vi "get tag counts.vi"(11 "data dictionary in":refnum<class "data dictionary.lvclass">) -> (2 "counts":T1[](array[typedef]), 3 "data dictionary out":refnum<class "data dictionary.lvclass">)   [LabVIEW 2013, in "tag bus.lvlib" / "data dictionary.lvclass"]
doc: "Gets the constitution of the data table, returning an array of types and the associated tag count of each type. If the dictionary is empty, this returns an empty array."
uses:
  data dictionary.lvclass
  table/allocation specification.ctl
  tag/Data Type.ctl
  data dictionary.lvclass/data dictionary.ctl
  tag/count types.vi
  tag/index to type.vi
  tag/tag descriptor.lvclass
  table/data table.lvlib
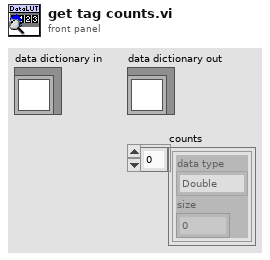
[diagram p1: front panel]
types:
  T1 = typedef "tag bus.lvlib/data table.lvlib/allocation specification.ctl" = cluster{"data type":T2, "size":i32}
  T2 = typedef "tag bus.lvlib/tag descriptor.lvclass/Data Type.ctl" = enum16{"Double", "Single", "I64", "I32", "I16", "I8", "U64", "U32", "U16", "U8", "Boolean", "String", "Array of Double", "Array of Single", "Array of I64", "Array of I32", "Array of I16", "Array of I8", "Array of U64", "Array of U32", "Array of U16", "Array of U8", "Array of Boolean", "Array of String"}
  T3 = typedef "tag bus.lvlib/binary search.lvlib/sorted list.ctl" = cluster{"sorted strings":string[], "sorted indices":i32[]}
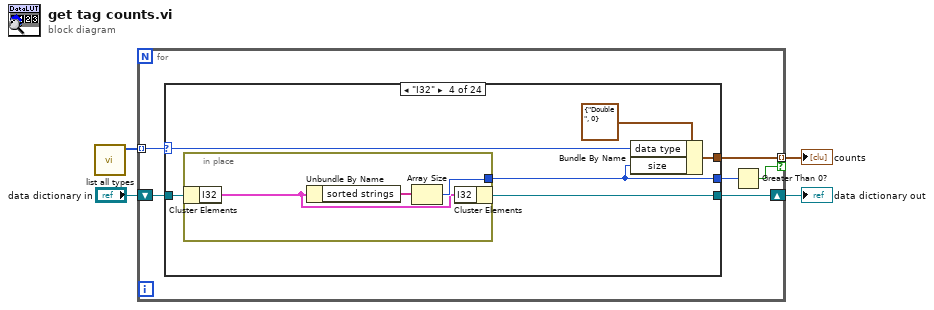
[diagram p0: block diagram]
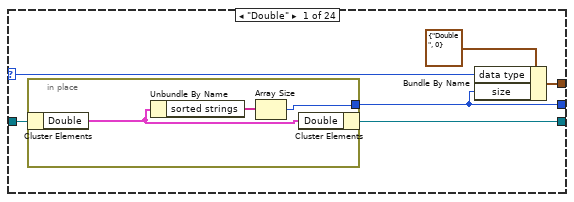
[diagram p2: hidden frame]
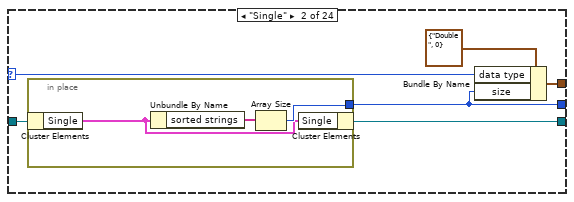
[diagram p3: hidden frame]
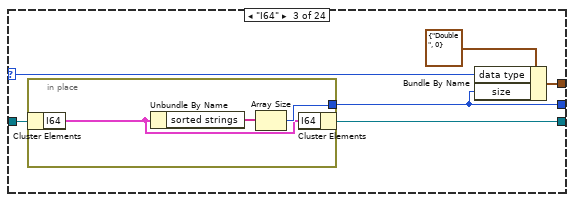
[diagram p4: hidden frame]
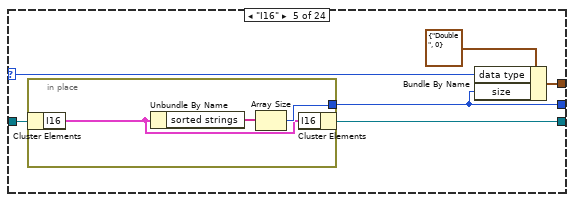
[diagram p5: hidden frame]
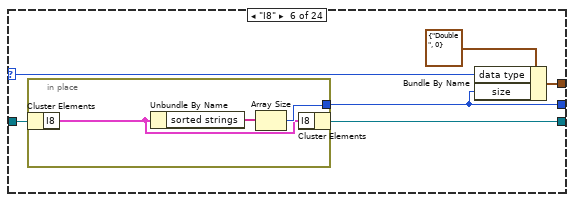
[diagram p6: hidden frame]
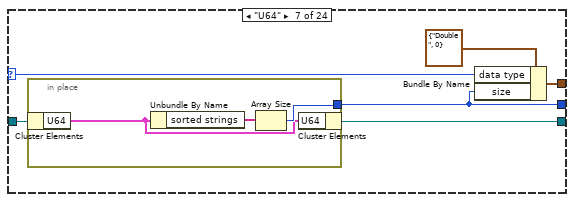
[diagram p7: hidden frame]
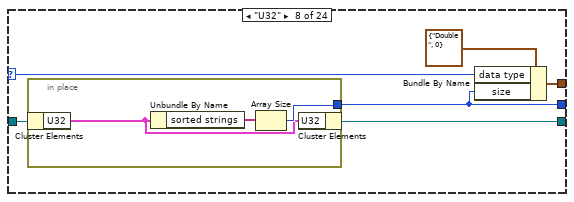
[diagram p8: hidden frame]
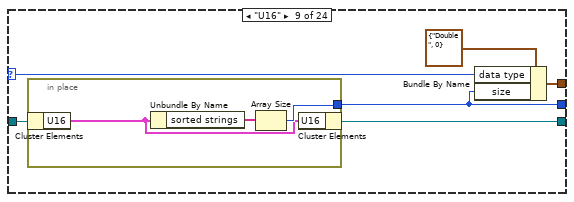
[diagram p9: hidden frame]
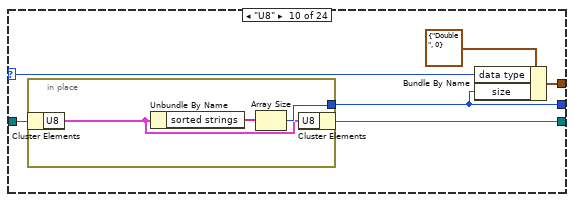
[diagram p10: hidden frame]
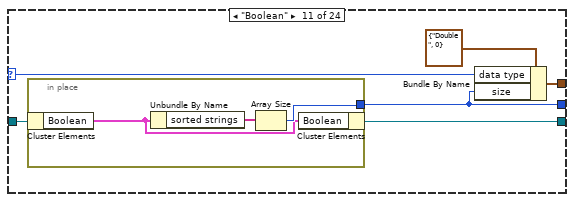
[diagram p11: hidden frame]
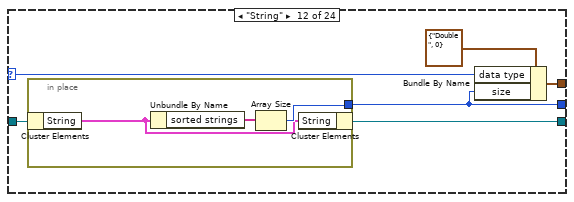
[diagram p12: hidden frame]
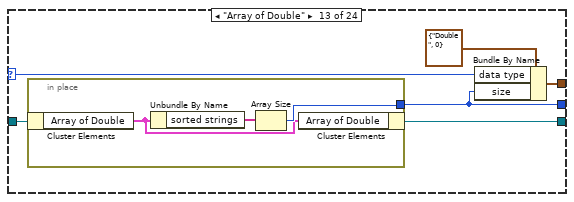
[diagram p13: hidden frame]
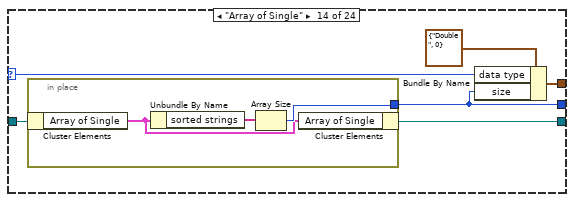
[diagram p14: hidden frame]
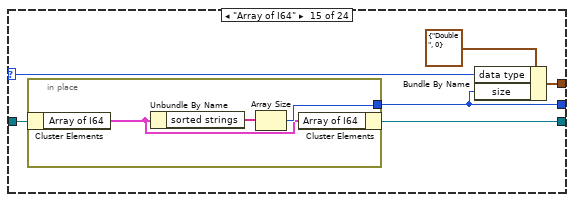
[diagram p15: hidden frame]
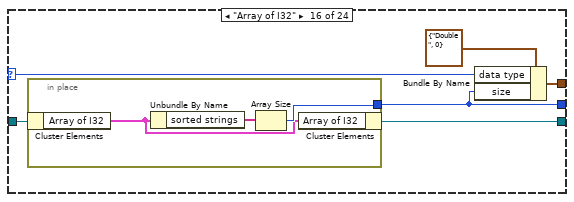
[diagram p16: hidden frame]
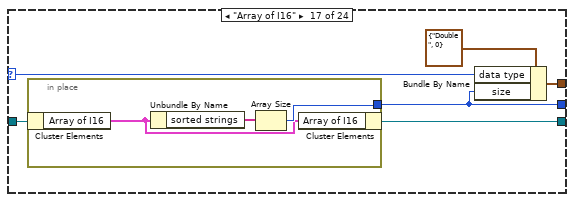
[diagram p17: hidden frame]
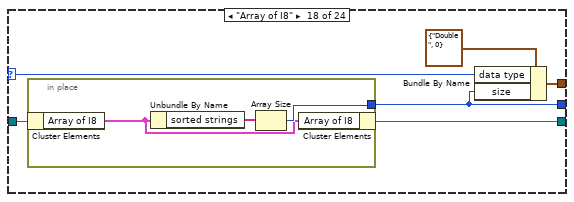
[diagram p18: hidden frame]
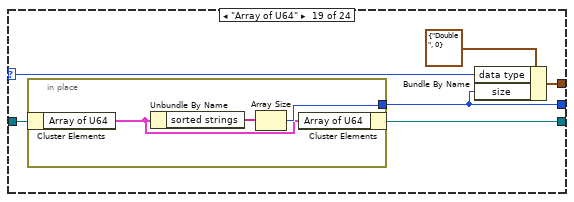
[diagram p19: hidden frame]
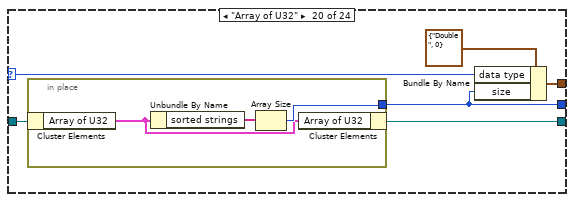
[diagram p20: hidden frame]
diagram:
  n1 = call "list all types.vi"() -> ("all types"=w3:T2[])  [unwired: 11 in]
  n2 = for {
    shift-right: [w8] -> w2
    shift-left: "data dictionary in" -> [w9]
    tunnel: w3 -> [w10] mode=indexing
    tunnel: [w7] -> w4 mode=indexing if=w6
    n3 = case shown="\"I32\"" w10 {
      selector: w10 -> [w13 w22 w31 w40 w49 w58 w67 w76 w85 w94 w103 w112 w121 w130 w139 w148 w157 w166 w175 w184 w193 w202 w211 w220]
      tunnel: w9 -> [w16 w25 w34 w43 w52 w61 w70 w79 w88 w97 w106 w115 w124 w133 w142 w151 w160 w169 w178 w187 w196 w205 w214 w223]
      tunnel: [w15 w24 w33 w42 w51 w60 w69 w78 w87 w96 w105 w114 w123 w132 w141 w150 w159 w168 w177 w186 w195 w204 w213 w222] -> w8
      tunnel: [w12 w21 w30 w39 w48 w57 w66 w75 w84 w93 w102 w111 w120 w129 w138 w147 w156 w165 w174 w183 w192 w201 w210 w219] -> w7
      tunnel: [w11 w20 w29 w38 w47 w56 w65 w74 w83 w92 w101 w110 w119 w128 w137 w146 w155 w164 w173 w182 w191 w200 w209 w218] -> w5
      frame "Double" {
        n4 = in-place {
          in-place-border: [w19] -> w11
          n5 = in-place-cluster #1(w16) -> ("Double"=w18:T3)
          n6 = Unbundle By Name(w18) -> ("sorted strings"=w17:string[])
          n7 = Array Size(array=w17) -> (size(s)=w19:i32)
          n8 = in-place-cluster #1("Double"=w18) -> (w15:refnum<class "data dictionary.lvclass">)
        }
        n9 = Bundle By Name(cluster=T1 {"data type"=enum."Double", "size"=0} ("allocation"), "data type"=w13, "size"=w11) -> (w12:T1)
      }
      frame "Single" {
        n10 = in-place {
          in-place-border: [w28] -> w20
          n11 = in-place-cluster #2(w25) -> ("Single"=w27:T3)
          n12 = Unbundle By Name(w27) -> ("sorted strings"=w26:string[])
          n13 = Array Size(array=w26) -> (size(s)=w28:i32)
          n14 = in-place-cluster #2("Single"=w27) -> (w24:refnum<class "data dictionary.lvclass">)
        }
        n15 = Bundle By Name(cluster=T1 {"data type"=enum."Double", "size"=0} ("allocation"), "data type"=w22, "size"=w20) -> (w21:T1)
      }
      frame "I64" {
        n16 = in-place {
          in-place-border: [w37] -> w29
          n17 = in-place-cluster #3(w34) -> ("I64"=w36:T3)
          n18 = Unbundle By Name(w36) -> ("sorted strings"=w35:string[])
          n19 = Array Size(array=w35) -> (size(s)=w37:i32)
          n20 = in-place-cluster #3("I64"=w36) -> (w33:refnum<class "data dictionary.lvclass">)
        }
        n21 = Bundle By Name(cluster=T1 {"data type"=enum."Double", "size"=0} ("allocation"), "data type"=w31, "size"=w29) -> (w30:T1)
      }
      frame "I32" {
        n22 = in-place {
          in-place-border: [w46] -> w38
          n23 = in-place-cluster #4(w43) -> ("I32"=w45:T3)
          n24 = Unbundle By Name(w45) -> ("sorted strings"=w44:string[])
          n25 = Array Size(array=w44) -> (size(s)=w46:i32)
          n26 = in-place-cluster #4("I32"=w45) -> (w42:refnum<class "data dictionary.lvclass">)
        }
        n27 = Bundle By Name(cluster=T1 {"data type"=enum."Double", "size"=0} ("allocation"), "data type"=w40, "size"=w38) -> (w39:T1)
      }
      frame "I16" {
        n28 = in-place {
          in-place-border: [w55] -> w47
          n29 = in-place-cluster #5(w52) -> ("I16"=w54:T3)
          n30 = Unbundle By Name(w54) -> ("sorted strings"=w53:string[])
          n31 = Array Size(array=w53) -> (size(s)=w55:i32)
          n32 = in-place-cluster #5("I16"=w54) -> (w51:refnum<class "data dictionary.lvclass">)
        }
        n33 = Bundle By Name(cluster=T1 {"data type"=enum."Double", "size"=0} ("allocation"), "data type"=w49, "size"=w47) -> (w48:T1)
      }
      frame "I8" {
        n34 = in-place {
          in-place-border: [w64] -> w56
          n35 = in-place-cluster #6(w61) -> ("I8"=w63:T3)
          n36 = Unbundle By Name(w63) -> ("sorted strings"=w62:string[])
          n37 = Array Size(array=w62) -> (size(s)=w64:i32)
          n38 = in-place-cluster #6("I8"=w63) -> (w60:refnum<class "data dictionary.lvclass">)
        }
        n39 = Bundle By Name(cluster=T1 {"data type"=enum."Double", "size"=0} ("allocation"), "data type"=w58, "size"=w56) -> (w57:T1)
      }
      frame "U64" {
        n40 = in-place {
          in-place-border: [w73] -> w65
          n41 = in-place-cluster #7(w70) -> ("U64"=w72:T3)
          n42 = Unbundle By Name(w72) -> ("sorted strings"=w71:string[])
          n43 = Array Size(array=w71) -> (size(s)=w73:i32)
          n44 = in-place-cluster #7("U64"=w72) -> (w69:refnum<class "data dictionary.lvclass">)
        }
        n45 = Bundle By Name(cluster=T1 {"data type"=enum."Double", "size"=0} ("allocation"), "data type"=w67, "size"=w65) -> (w66:T1)
      }
      frame "U32" {
        n46 = in-place {
          in-place-border: [w82] -> w74
          n47 = in-place-cluster #8(w79) -> ("U32"=w81:T3)
          n48 = Unbundle By Name(w81) -> ("sorted strings"=w80:string[])
          n49 = Array Size(array=w80) -> (size(s)=w82:i32)
          n50 = in-place-cluster #8("U32"=w81) -> (w78:refnum<class "data dictionary.lvclass">)
        }
        n51 = Bundle By Name(cluster=T1 {"data type"=enum."Double", "size"=0} ("allocation"), "data type"=w76, "size"=w74) -> (w75:T1)
      }
      frame "U16" {
        n52 = in-place {
          in-place-border: [w91] -> w83
          n53 = in-place-cluster #9(w88) -> ("U16"=w90:T3)
          n54 = Unbundle By Name(w90) -> ("sorted strings"=w89:string[])
          n55 = Array Size(array=w89) -> (size(s)=w91:i32)
          n56 = in-place-cluster #9("U16"=w90) -> (w87:refnum<class "data dictionary.lvclass">)
        }
        n57 = Bundle By Name(cluster=T1 {"data type"=enum."Double", "size"=0} ("allocation"), "data type"=w85, "size"=w83) -> (w84:T1)
      }
      frame "U8" {
        n58 = in-place {
          in-place-border: [w100] -> w92
          n59 = in-place-cluster #10(w97) -> ("U8"=w99:T3)
          n60 = Unbundle By Name(w99) -> ("sorted strings"=w98:string[])
          n61 = Array Size(array=w98) -> (size(s)=w100:i32)
          n62 = in-place-cluster #10("U8"=w99) -> (w96:refnum<class "data dictionary.lvclass">)
        }
        n63 = Bundle By Name(cluster=T1 {"data type"=enum."Double", "size"=0} ("allocation"), "data type"=w94, "size"=w92) -> (w93:T1)
      }
      frame "Boolean" {
        n64 = in-place {
          in-place-border: [w109] -> w101
          n65 = in-place-cluster #11(w106) -> ("Boolean"=w108:T3)
          n66 = Unbundle By Name(w108) -> ("sorted strings"=w107:string[])
          n67 = Array Size(array=w107) -> (size(s)=w109:i32)
          n68 = in-place-cluster #11("Boolean"=w108) -> (w105:refnum<class "data dictionary.lvclass">)
        }
        n69 = Bundle By Name(cluster=T1 {"data type"=enum."Double", "size"=0} ("allocation"), "data type"=w103, "size"=w101) -> (w102:T1)
      }
      frame "String" {
        n70 = in-place {
          in-place-border: [w118] -> w110
          n71 = in-place-cluster #12(w115) -> ("String"=w117:T3)
          n72 = Unbundle By Name(w117) -> ("sorted strings"=w116:string[])
          n73 = Array Size(array=w116) -> (size(s)=w118:i32)
          n74 = in-place-cluster #12("String"=w117) -> (w114:refnum<class "data dictionary.lvclass">)
        }
        n75 = Bundle By Name(cluster=T1 {"data type"=enum."Double", "size"=0} ("allocation"), "data type"=w112, "size"=w110) -> (w111:T1)
      }
      frame "Array of Double" {
        n76 = in-place {
          in-place-border: [w127] -> w119
          n77 = in-place-cluster #13(w124) -> ("Array of Double"=w126:T3)
          n78 = Unbundle By Name(w126) -> ("sorted strings"=w125:string[])
          n79 = Array Size(array=w125) -> (size(s)=w127:i32)
          n80 = in-place-cluster #13("Array of Double"=w126) -> (w123:refnum<class "data dictionary.lvclass">)
        }
        n81 = Bundle By Name(cluster=T1 {"data type"=enum."Double", "size"=0} ("allocation"), "data type"=w121, "size"=w119) -> (w120:T1)
      }
      frame "Array of Single" {
        n82 = in-place {
          in-place-border: [w136] -> w128
          n83 = in-place-cluster #14(w133) -> ("Array of Single"=w135:T3)
          n84 = Unbundle By Name(w135) -> ("sorted strings"=w134:string[])
          n85 = Array Size(array=w134) -> (size(s)=w136:i32)
          n86 = in-place-cluster #14("Array of Single"=w135) -> (w132:refnum<class "data dictionary.lvclass">)
        }
        n87 = Bundle By Name(cluster=T1 {"data type"=enum."Double", "size"=0} ("allocation"), "data type"=w130, "size"=w128) -> (w129:T1)
      }
      frame "Array of I64" {
        n88 = in-place {
          in-place-border: [w145] -> w137
          n89 = in-place-cluster #15(w142) -> ("Array of I64"=w144:T3)
          n90 = Unbundle By Name(w144) -> ("sorted strings"=w143:string[])
          n91 = Array Size(array=w143) -> (size(s)=w145:i32)
          n92 = in-place-cluster #15("Array of I64"=w144) -> (w141:refnum<class "data dictionary.lvclass">)
        }
        n93 = Bundle By Name(cluster=T1 {"data type"=enum."Double", "size"=0} ("allocation"), "data type"=w139, "size"=w137) -> (w138:T1)
      }
      frame "Array of I32" {
        n94 = in-place {
          in-place-border: [w154] -> w146
          n95 = in-place-cluster #16(w151) -> ("Array of I32"=w153:T3)
          n96 = Unbundle By Name(w153) -> ("sorted strings"=w152:string[])
          n97 = Array Size(array=w152) -> (size(s)=w154:i32)
          n98 = in-place-cluster #16("Array of I32"=w153) -> (w150:refnum<class "data dictionary.lvclass">)
        }
        n99 = Bundle By Name(cluster=T1 {"data type"=enum."Double", "size"=0} ("allocation"), "data type"=w148, "size"=w146) -> (w147:T1)
      }
      frame "Array of I16" {
        n100 = in-place {
          in-place-border: [w163] -> w155
          n101 = in-place-cluster #17(w160) -> ("Array of I16"=w162:T3)
          n102 = Unbundle By Name(w162) -> ("sorted strings"=w161:string[])
          n103 = Array Size(array=w161) -> (size(s)=w163:i32)
          n104 = in-place-cluster #17("Array of I16"=w162) -> (w159:refnum<class "data dictionary.lvclass">)
        }
        n105 = Bundle By Name(cluster=T1 {"data type"=enum."Double", "size"=0} ("allocation"), "data type"=w157, "size"=w155) -> (w156:T1)
      }
      frame "Array of I8" {
        n106 = in-place {
          in-place-border: [w172] -> w164
          n107 = in-place-cluster #18(w169) -> ("Array of I8"=w171:T3)
          n108 = Unbundle By Name(w171) -> ("sorted strings"=w170:string[])
          n109 = Array Size(array=w170) -> (size(s)=w172:i32)
          n110 = in-place-cluster #18("Array of I8"=w171) -> (w168:refnum<class "data dictionary.lvclass">)
        }
        n111 = Bundle By Name(cluster=T1 {"data type"=enum."Double", "size"=0} ("allocation"), "data type"=w166, "size"=w164) -> (w165:T1)
      }
      frame "Array of U64" {
        n112 = in-place {
          in-place-border: [w181] -> w173
          n113 = in-place-cluster #19(w178) -> ("Array of U64"=w180:T3)
          n114 = Unbundle By Name(w180) -> ("sorted strings"=w179:string[])
          n115 = Array Size(array=w179) -> (size(s)=w181:i32)
          n116 = in-place-cluster #19("Array of U64"=w180) -> (w177:refnum<class "data dictionary.lvclass">)
        }
        n117 = Bundle By Name(cluster=T1 {"data type"=enum."Double", "size"=0} ("allocation"), "data type"=w175, "size"=w173) -> (w174:T1)
      }
      frame "Array of U32" {
        n118 = in-place {
          in-place-border: [w190] -> w182
          n119 = in-place-cluster #20(w187) -> ("Array of U32"=w189:T3)
          n120 = Unbundle By Name(w189) -> ("sorted strings"=w188:string[])
          n121 = Array Size(array=w188) -> (size(s)=w190:i32)
          n122 = in-place-cluster #20("Array of U32"=w189) -> (w186:refnum<class "data dictionary.lvclass">)
        }
        n123 = Bundle By Name(cluster=T1 {"data type"=enum."Double", "size"=0} ("allocation"), "data type"=w184, "size"=w182) -> (w183:T1)
      }
      frame "Array of U16" {
        n124 = in-place {
          in-place-border: [w199] -> w191
          n125 = in-place-cluster #21(w196) -> ("Array of U16"=w198:T3)
          n126 = Unbundle By Name(w198) -> ("sorted strings"=w197:string[])
          n127 = Array Size(array=w197) -> (size(s)=w199:i32)
          n128 = in-place-cluster #21("Array of U16"=w198) -> (w195:refnum<class "data dictionary.lvclass">)
        }
        n129 = Bundle By Name(cluster=T1 {"data type"=enum."Double", "size"=0} ("allocation"), "data type"=w193, "size"=w191) -> (w192:T1)
      }
      frame "Array of U8" {
        n130 = in-place {
          in-place-border: [w208] -> w200
          n131 = in-place-cluster #22(w205) -> ("Array of U8"=w207:T3)
          n132 = Unbundle By Name(w207) -> ("sorted strings"=w206:string[])
          n133 = Array Size(array=w206) -> (size(s)=w208:i32)
          n134 = in-place-cluster #22("Array of U8"=w207) -> (w204:refnum<class "data dictionary.lvclass">)
        }
        n135 = Bundle By Name(cluster=T1 {"data type"=enum."Double", "size"=0} ("allocation"), "data type"=w202, "size"=w200) -> (w201:T1)
      }
      frame "Array of Boolean" {
        n136 = in-place {
          in-place-border: [w217] -> w209
          n137 = in-place-cluster #23(w214) -> ("Array of Boolean"=w216:T3)
          n138 = Unbundle By Name(w216) -> ("sorted strings"=w215:string[])
          n139 = Array Size(array=w215) -> (size(s)=w217:i32)
          n140 = in-place-cluster #23("Array of Boolean"=w216) -> (w213:refnum<class "data dictionary.lvclass">)
        }
        n141 = Bundle By Name(cluster=T1 {"data type"=enum."Double", "size"=0} ("allocation"), "data type"=w211, "size"=w209) -> (w210:T1)
      }
      frame "Array of String" {
        n142 = in-place {
          in-place-border: [w226] -> w218
          n143 = in-place-cluster #24(w223) -> ("Array of String"=w225:T3)
          n144 = Unbundle By Name(w225) -> ("sorted strings"=w224:string[])
          n145 = Array Size(array=w224) -> (size(s)=w226:i32)
          n146 = in-place-cluster #24("Array of String"=w225) -> (w222:refnum<class "data dictionary.lvclass">)
        }
        n147 = Bundle By Name(cluster=T1 {"data type"=enum."Double", "size"=0} ("allocation"), "data type"=w220, "size"=w218) -> (w219:T1)
      }
    }
    n148 = Greater Than 0?(x=w5) -> (x > 0?=w6:bool)
  }
  "counts" <- w4
  "data dictionary out" <- w2
